vi "Add Key.vi"(0 "refnum":T1, 1 "section":string, 5 "key":string, 7 "value":string, 11 "error in (no error)":errorcluster, 12 "add comment":bool=TRUE) -> (4 "refnum out":T1, 6 "key exists?":bool, 15 "error out":errorcluster)   [LabVIEW 2020, in "NI_LVConfig.lvlib"]
uses:
  NI_LVConfig.lvlib
  Config Data RefNum.ctl
  Section.ctl
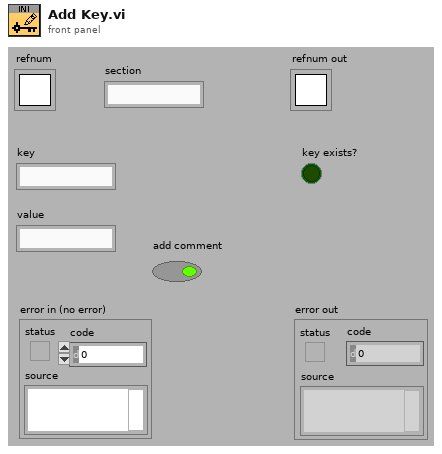
[diagram p1: front panel]
types:
  T1 = typedef "NI_LVConfig.lvlib/Config Data RefNum.ctl" = refnum<k1>
  T2 = typedef "NI_LVConfig.lvlib/Section.ctl" = cluster{"name":string, "comment":string, "kvc":string[][]}
  T3 = typedef "NI_LVConfig.lvlib/Config Queue.ctl" = refnum<queue>
  T4 = typedef "NI_LVConfig.lvlib/Config Data.ctl" = cluster{"sections":T2[], "path":path, "dirty":bool}
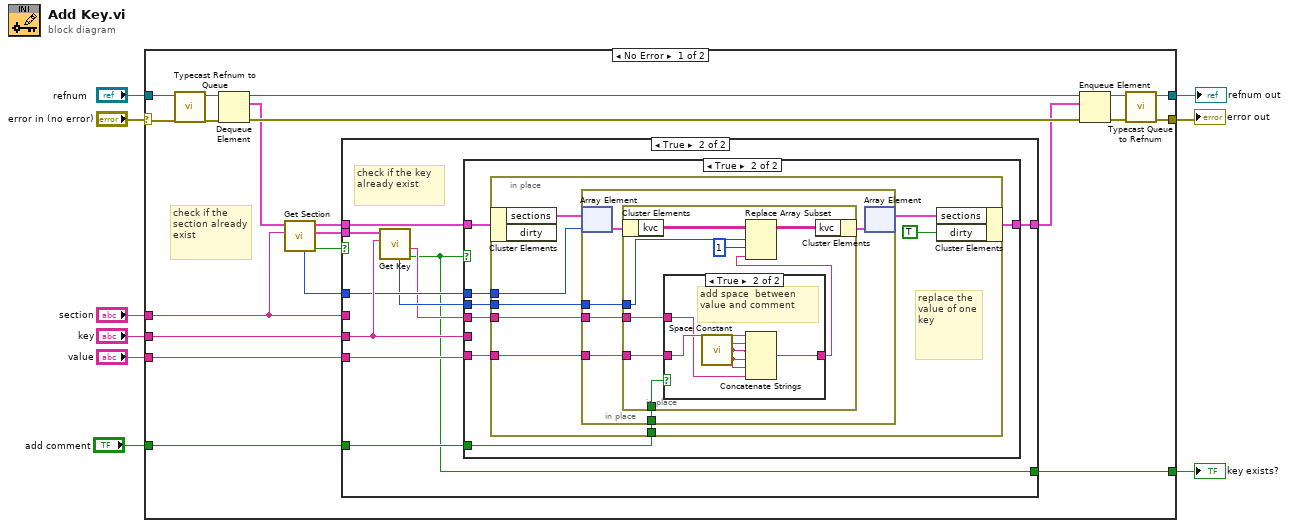
[diagram p0: block diagram]
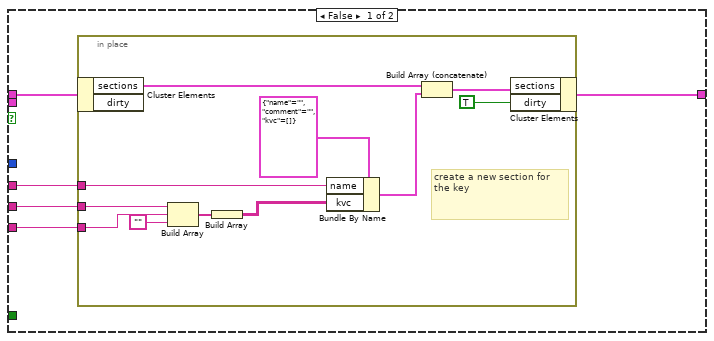
[diagram p2: hidden frame]
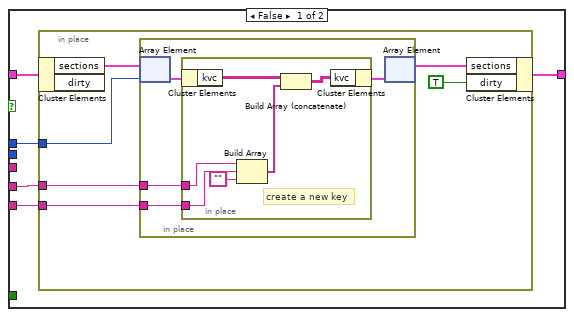
[diagram p3: hidden frame]
diagram:
  n1 = case shown="No Error" "error in (no error)" {
    selector: "error in (no error)" -> [w17 w111]
    tunnel: [w24 w111] -> w8
    tunnel: [w21 w110] -> w2
    tunnel: "refnum" -> [w23 w110]
    tunnel: "section" -> [w14 _]
    tunnel: "key" -> [w28 _]
    tunnel: "value" -> [w27 _]
    tunnel: [w10 _] -> w4
    tunnel: "add comment" -> [w20 _]
    frame No Error {
      # "check if the section already exist"
      n2 = call "Typecast Refnum to Queue.vi"("refnum in"=w23) -> ("queue out"=w18:T3)  [unwired: 10 out]
      n3 = Dequeue Element(queue=w18, error in (no error)=w17) -> (queue out=w26:T3, element=w16:T4, error out=w25:errorcluster)  [unwired: 2 out]
      n4 = call "Get Section.vi"("section"=w14, "element"=w16) -> ("section exists?"=w13:bool, "section data"=w12:T2, "element out"=w15:T4, "section index"=w11:i32)  [unwired: 6 out]
      n5 = case shown="True" w13 {
        tunnel: w15 -> [w32 w54]
        tunnel: w28 -> [w31 w49]
        tunnel: w27 -> [w30 w53]
        tunnel: [w29 w52] -> w19
        tunnel: w14 -> [w33 _]
        tunnel: w20 -> [_ w51]
        tunnel: w12 -> [_ w50]
        tunnel: w11 -> [_ w48]
        tunnel: [_ w45] -> w10
        frame False {
          n6 = in-place "In Place Element Structure" {
            in-place-border: w30 -> [w43]
            in-place-border: w31 -> [w44]
            in-place-border: w33 -> [w41]
            # "create a new section for the key"
            n7 = in-place-cluster #1(w32) -> ("sections"=w42:T2[])  [unwired: 1 out]
            n8 = Build Array(w44, w43, "") -> (w39:string[])
            n9 = Build Array(w39) -> (w34:string[][])
            n10 = Bundle By Name(cluster=T2 {"name"="", "comment"="", "kvc"=[]} ("Section"), "name"=w41, "kvc"=w34) -> (w40:T2)
            n11 = Build Array (concatenate)(w42, w40) -> (w38:T2[])
            n12 = in-place-cluster #1("sections"=w38, "dirty"=TRUE) -> (w29:T4)
          }
        }
        frame True {
          # "check if the key already exist"
          n13 = call "Get Key.vi"("key"=w49, "section data"=w50) -> ("key exists?"=w45:bool, "comment"=w46:string, "key index"=w47:i32)  [unwired: 7 out]
          n14 = case shown="True" w45 {
            tunnel: w47 -> [_ w80]
            tunnel: w54 -> [w59 w82]
            tunnel: w48 -> [w58 w81]
            tunnel: w53 -> [w57 w79]
            tunnel: [w55 w78] -> w52
            tunnel: w49 -> [w56 _]
            tunnel: w51 -> [_ w76]
            tunnel: w46 -> [_ w77]
            frame False {
              n15 = in-place "In Place Element Structure" {
                in-place-border: w58 -> [w64]
                in-place-border: w57 -> [w63]
                in-place-border: w56 -> [w62]
                n16 = in-place-cluster #2(w59) -> ("sections"=w65:T2[])  [unwired: 1 out]
                n17 = in-place "In Place Element Structure" {
                  in-place-border: w63 -> [w67]
                  in-place-border: w62 -> [w66]
                  n18 = in-place-array #3(w65, w64) -> (w69:T2)
                  n19 = in-place "In Place Element Structure" {
                    in-place-border: w67 -> [w72]
                    in-place-border: w66 -> [w71]
                    # "create a new key"
                    n20 = in-place-cluster #4(w69) -> ("kvc"=w75:string[][])
                    n21 = Build Array(w71, w72, "") -> (w73:string[])
                    n22 = Build Array (concatenate)(w75, w73) -> (w74:string[][])
                    n23 = in-place-cluster #4("kvc"=w74) -> (w68:T2)
                  }
                  n24 = in-place-array #3(w68) -> (w61:T2[])  [unwired: 1 out]
                }
                n25 = in-place-cluster #2("sections"=w61, "dirty"=TRUE) -> (w55:T4)
              }
            }
            frame True {
              n26 = in-place "In Place Element Structure" {
                in-place-border: w81 -> [w89]
                in-place-border: w80 -> [w88]
                in-place-border: w79 -> [w87]
                in-place-border: w77 -> [w85]
                in-place-border: w76 -> [w84]
                # "replace the value of one key"
                n27 = in-place-cluster #5(w82) -> ("sections"=w90:T2[])  [unwired: 1 out]
                n28 = in-place "In Place Element Structure" {
                  in-place-border: w88 -> [w95]
                  in-place-border: w87 -> [w94]
                  in-place-border: w85 -> [w92]
                  in-place-border: w84 -> [w91]
                  n29 = in-place-array #6(w90, w89) -> (w96:T2)
                  n30 = in-place "In Place Element Structure" {
                    in-place-border: w95 -> [w102]
                    in-place-border: w94 -> [w100]
                    in-place-border: w92 -> [w99]
                    in-place-border: w91 -> [w98]
                    n31 = in-place-cluster #7(w96) -> ("kvc"=w104:string[][])
                    n32 = case shown="True" w98 {
                      tunnel: w100 -> [w105 w109]
                      tunnel: w99 -> [_ w107]
                      tunnel: [w105 w108] -> w97
                      frame False {
                      }
                      frame True {
                        # "add space  between value and comment"
                        n33 = call "Space Constant.vi"() -> ("String"=w106:string)
                        n34 = Concatenate Strings(w109, w106, w106, w106, w106, w107) -> (w108:string)
                      }
                    }
                    n35 = Replace Array Subset(array=w104, new element=w97, index (row)=w102, index (col)=1 ("disabled index (col)")) -> (w103:string[][])
                    n36 = in-place-cluster #7("kvc"=w103) -> (w93:T2)
                  }
                  n37 = in-place-array #6(w93) -> (w86:T2[])  [unwired: 1 out]
                }
                n38 = in-place-cluster #5("sections"=w86, "dirty"=TRUE) -> (w78:T4)
              }
            }
          }
        }
      }
      n39 = Enqueue Element(queue=w26, element=w19, error in (no error)=w25) -> (queue out=w22:T3, error out=w24:errorcluster)  [unwired: 2 out]
      n40 = call "Typecast Queue to Refnum.vi"("queue in"=w22) -> ("refnum out"=w21:T1)  [unwired: 10 out]
    }
    frame Error {
    }
  }
  "error out" <- w8
  "key exists?" <- w4
  "refnum out" <- w2
